vi "Process.vi"(8 "error in (no error)":errorcluster, 11 "qbus in":refnum<class "Qbus.lvclass">) -> (0 "error out":errorcluster)   [LabVIEW 2017, in "TraceLogger.lvlib"]
doc: "This process receives tracepoint instances, writes them to temporary log files on the device disk, and forwards them to the TracePoint Synchronizer process. Separately, the TracePoint Synchronizer process sends tracepoint instances to NI InsightCM Server and informs Tracelogger process when the list of enabled tracepoints changes."
uses:
  <vilib>/addons/TraceLogger/TraceLogger.lvlib
  <vilib>/addons/Qbus/Qbus.lvclass
  <vilib>/addons/TraceLogger/controls/config.ctl
  <vilib>/addons/TraceLogger/controls/LogTracepoint.ctl
  <vilib>/addons/TimerProcess/controls/taskType.ctl
  <vilib>/addons/TimerProcess/TimerProcess.lvlib
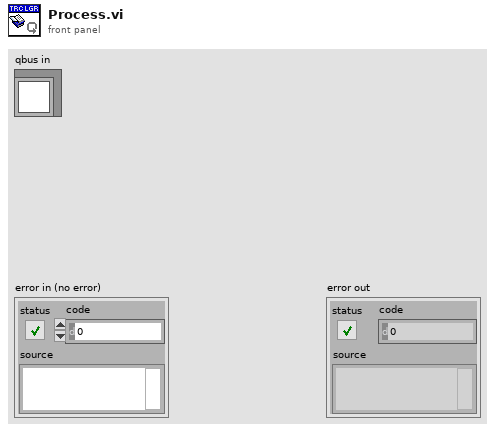
[diagram p1: front panel]
types:
  T1 = typedef "TraceLogger.lvlib/config.ctl" = cluster{"log dir":path, "tracepoints dir":path, "BufferQ":refnum<queue>}
  T2 = typedef "TraceLogger.lvlib/LogTracepoint.ctl" = cluster{"tracepoint":string, "log string":string}
  T3 = typedef "TimerProcess.lvlib/taskType.ctl" = enum16{"single", "repeat"}
  T4 = typedef "TracpointDirectories.ctl" = cluster{"log directory":path, "tracpoint directory":path}
  T5 = typedef "TraceLogger.lvlib/TracepointConfig.ctl" = cluster{"name":string, "enabled":bool}
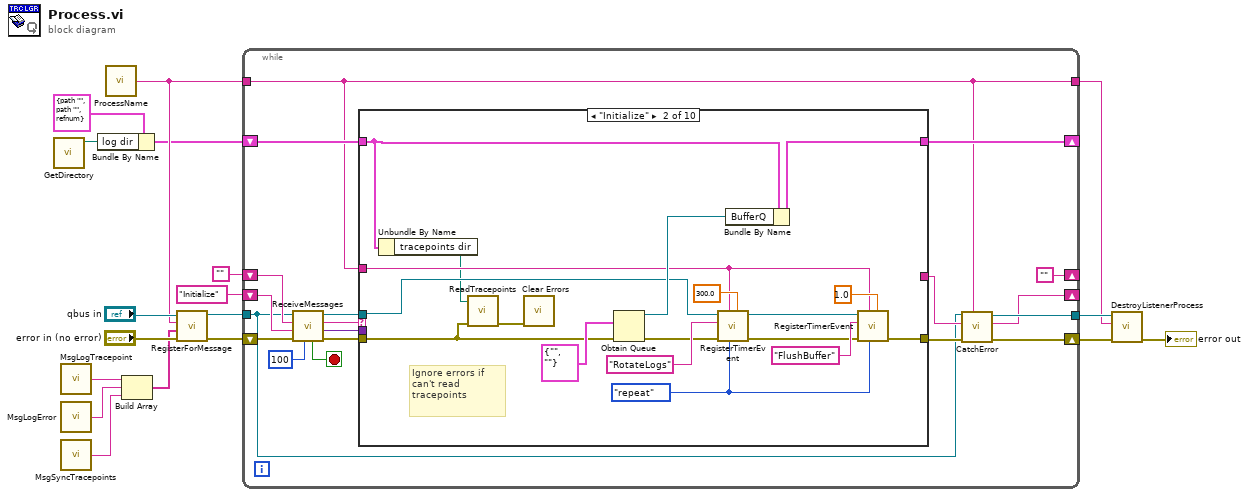
[diagram p0: block diagram]
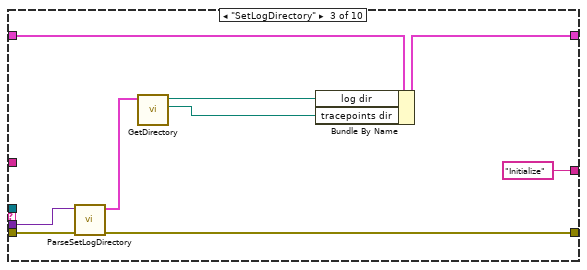
[diagram p3: hidden frame]
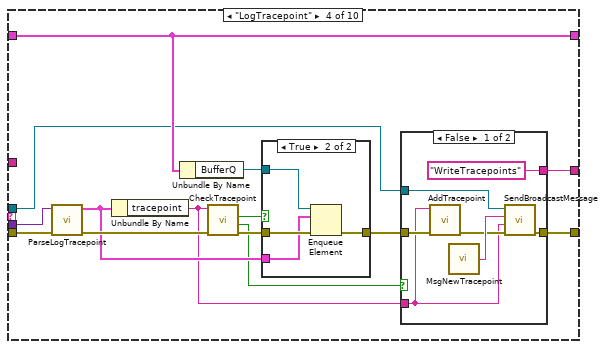
[diagram p4: hidden frame]
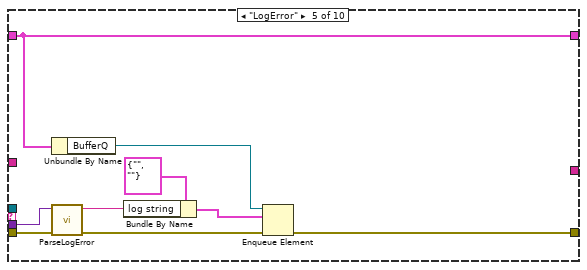
[diagram p7: hidden frame]
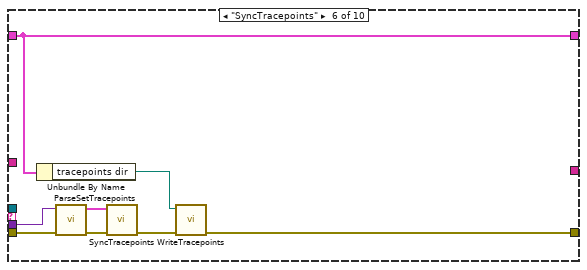
[diagram p8: hidden frame]
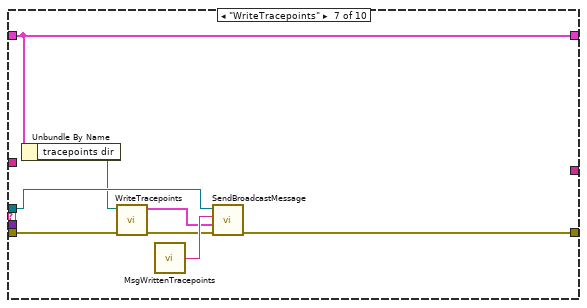
[diagram p9: hidden frame]
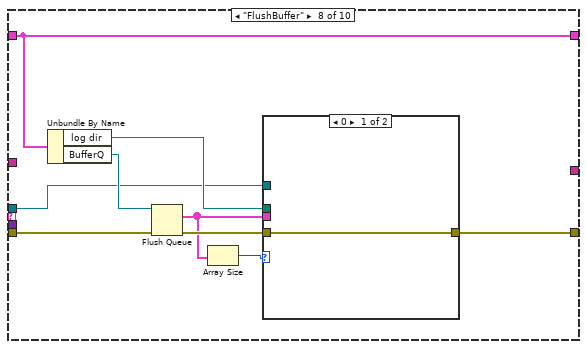
[diagram p10: hidden frame]
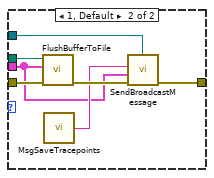
[diagram p11: hidden frame]
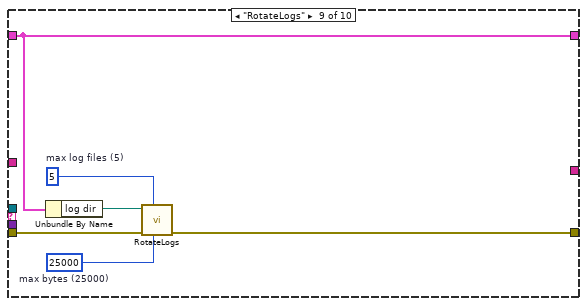
[diagram p12: hidden frame]
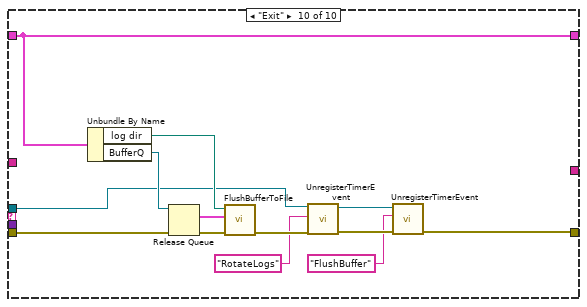
[diagram p13: hidden frame]
diagram:
  n1 = call <vilib>:"GetDirectory.vi"() -> ("log directory"=w4:path)  [unwired: 10 in, 1 out]
  n2 = call <vilib>:"MsgLogTracepoint.vi"() -> ("message name"=w2:string)  [unwired: 5 in]
  n3 = call <vilib>:"MsgLogError.vi"() -> ("message name"=w1:string)  [unwired: 5 in]
  n4 = call <vilib>:"MsgSyncTracepoints.vi"() -> ("message name"=w3:string)  [unwired: 5 in]
  n5 = Bundle By Name(cluster=T1 {"log dir"=path "", "tracepoints dir"=path "", "BufferQ"=refnum} ("config"), "log dir"=w4) -> (w5:T1)
  n6 = call <vilib>:"ProcessName.vi"() -> ("process name"=w8:string)  [unwired: 5 in]
  n7 = Build Array(w2, w1, w3) -> (w7:string[])
  n8 = call <vilib>:"RegisterForMessage.vi"("error in (no error)"="error in (no error)", "message names"=w7, "process name"=w8, "Qbus in"="qbus in") -> ("error in (no error)"=w17:errorcluster, "Qbus out"=w16:refnum<class "Qbus.lvclass">)  [unwired: 6 in]
  n9 = while {
    shift-right: [""] -> _
    shift-left: "" -> [w35]
    tunnel: w16 -> [w21]
    tunnel: w8 -> [w24]
    tunnel: [w26] -> w13
    tunnel: [w24] -> w12
    shift-right: [w25] -> _
    shift-left: "Initialize" -> [w30]
    shift-right: [w28] -> _
    shift-left: w5 -> [w29]
    shift-right: [w27] -> w15
    shift-left: w17 -> [w37]
    stop <- w36 stop-if-true
    n10 = call <vilib>:"ReceiveMessages.vi"("timeout(100)"=100, "error in (no error)"=w37, "priority action"=w30, "default action"=w35, "qbus in"=w21) -> ("error out"=w34:errorcluster, "message value"=w31:variant, "action"=w20:string, "qbus out"=w32:refnum<class "Qbus.lvclass">, "exit"=w36:bool)  [unwired: 2 in]
    n11 = case shown="\"Initialize\"" w20 {
      tunnel: w34 -> [w39 w42 w66 w80 w102 w110 w117 w126 w141 w151]
      tunnel: w32 -> [_ w43 _ w70 _ _ w114 w122 _ w145]
      tunnel: [w39 w45 w65 w69 w98 w103 w115 w121 w140 w146] -> w22
      tunnel: w31 -> [_ _ w64 w79 w101 w109 _ _ _ _]
      tunnel: w29 -> [w38 w41 w63 w77 w100 w106 w118 w127 w139 w150]
      tunnel: [w38 w55 w62 w77 w100 w106 w118 w127 w139 w150] -> w28
      tunnel: w24 -> [_ w44 _ _ _ _ _ _ _ _]
      tunnel: [_ _ "Initialize" w67 _ _ _ _ _ _] -> w23
      frame "", Default {
      }
      frame "Initialize" {
        w51 = taskType."repeat" ("type")
        # "Ignore errors if can't read tracepoints"
        n12 = Unbundle By Name(w41) -> ("tracepoints dir"=w40:path)
        n13 = call <vilib>:"ReadTracepoints.vi"("error in (no error)"=w42, "log dir"=w40) -> ("error out"=w57:errorcluster)  [unwired: 9 in]
        n14 = call <vilib>:"Clear Errors.vi"("error in (no error)"=w57) -> ()  [unwired: 5 in, 2 out]
        n15 = Obtain Queue(element data type=T2 {"tracepoint"="", "log string"=""} ("Buffer"), error in (no error)=w42) -> (queue out=w54:refnum<queue>, error out=w46:errorcluster)  [unwired: 3 in, 1 out]
        n16 = call <vilib>:"RegisterTimerEvent.vi"("interval (sec)"=300.0, "type"=w51, "process name"=w44, "error in (no error)"=w46, "callback action"="RotateLogs" ("CallBackLoop"), "qbus in"=w43) -> ("error out"=w49:errorcluster, "qbus out"=w53:refnum<class "Qbus.lvclass">)  [unwired: 4 in]
        n17 = Bundle By Name(cluster=w41, "BufferQ"=w54) -> (w55:T1)
        n18 = call <vilib>:"RegisterTimerEvent.vi"("interval (sec)"=1.0, "type"=w51, "process name"=w44, "error in (no error)"=w49, "callback action"="FlushBuffer" ("CallBackLoop"), "qbus in"=w53) -> ("error out"=w45:errorcluster)  [unwired: 4 in, 1 out]
      }
      frame "SetLogDirectory" {
        n19 = call <vilib>:"ParseSetLogDirectory.vi"("error in (no error)"=w66, "message body"=w64) -> ("error out"=w65:errorcluster, "tracepoint directories"=w60:T4)  [unwired: 8 in]
        n20 = call <vilib>:"GetDirectory.vi"("tracpoint directories"=w60) -> ("tracepoint directory"=w58:path, "log directory"=w59:path)  [unwired: 9 in]
        n21 = Bundle By Name(cluster=w63, "log dir"=w59, "tracepoints dir"=w58) -> (w62:T1)
      }
      frame "LogTracepoint" {
        n22 = call <vilib>:"ParseLogTracepoint.vi"("error in (no error)"=w80, "message body"=w79) -> ("error out"=w78:errorcluster, "tracelog"=w73:T2)  [unwired: 8 in]
        n23 = Unbundle By Name(w73) -> ("tracepoint"=w68:string)
        n24 = Unbundle By Name(w77) -> ("BufferQ"=w74:refnum<queue>)
        n25 = call <vilib>:"CheckTracepoint.vi"("error in (no error)"=w78, "tracepoint"=w68) -> ("error out"=w75:errorcluster, "found"=w71:bool, "enabled"=w76:bool)  [unwired: 7 in]
        n26 = case shown="True" w76 {
          tunnel: w75 -> [w89 w93]
          tunnel: w74 -> [_ w92]
          tunnel: w73 -> [_ w91]
          tunnel: [w89 w90] -> w72
          frame False {
          }
          frame True {
            n27 = Enqueue Element(queue=w92, element=w91, error in (no error)=w93) -> (error out=w90:errorcluster)  [unwired: 1 in, 2 out]
          }
        }
        n28 = case shown="False" w71 {
          tunnel: w72 -> [w83 w88]
          tunnel: w70 -> [w87 _]
          tunnel: [w85 w88] -> w69
          tunnel: w68 -> [w81 _]
          tunnel: ["WriteTracepoints" _] -> w67
          frame False {
            n29 = call <vilib>:"AddTracepoint.vi"("error in (no error)"=w83, "tracepoint"=w81) -> ("error out"=w82:errorcluster)  [unwired: 9 in]
            n30 = call <vilib>:"MsgNewTracepoint.vi"() -> ("message name"=w86:string)  [unwired: 5 in]
            n31 = call <vilib>:"SendBroadcastMessage.vi"("error in (no error)"=w82, "message value"=w81, "message name"=w86, "Qbus in"=w87) -> ("error in (no error)"=w85:errorcluster)  [unwired: 6 in, 1 out]
          }
          frame True {
          }
        }
      }
      frame "LogError" {
        n32 = Unbundle By Name(w100) -> ("BufferQ"=w99:refnum<queue>)
        n33 = call <vilib>:"ParseLogError.vi"("error in (no error)"=w102, "message body"=w101) -> ("error out"=w97:errorcluster, "error string"=w95:string)  [unwired: 8 in]
        n34 = Bundle By Name(cluster=T2 {"tracepoint"="", "log string"=""} ("element"), "log string"=w95) -> (w94:T2)
        n35 = Enqueue Element(queue=w99, element=w94, error in (no error)=w97) -> (error out=w98:errorcluster)  [unwired: 1 in, 2 out]
      }
      frame "SyncTracepoints" {
        n36 = Unbundle By Name(w106) -> ("tracepoints dir"=w105:path)
        n37 = call <vilib>:"ParseSetTracepoints.vi"("error in (no error)"=w110, "message body"=w109) -> ("error out"=w108:errorcluster, "tracepoints"=w107:T5[])  [unwired: 8 in]
        n38 = call <vilib>:"SyncTracepoints.vi"("error in (no error)"=w108, "new tracepoints"=w107) -> ("error out"=w104:errorcluster)  [unwired: 9 in]
        n39 = call <vilib>:"WriteTracepoints.vi"("error in (no error)"=w104, "log dir"=w105) -> ("error out"=w103:errorcluster)  [unwired: 8 in, 1 out]
      }
      frame "WriteTracepoints" {
        n40 = Unbundle By Name(w118) -> ("tracepoints dir"=w113:path)
        n41 = call <vilib>:"WriteTracepoints.vi"("error in (no error)"=w117, "log dir"=w113) -> ("error out"=w111:errorcluster, "tracepoints"=w112:T5[])  [unwired: 8 in]
        n42 = call <vilib>:"MsgWrittenTracepoints.vi"() -> ("message name"=w116:string)  [unwired: 5 in]
        n43 = call <vilib>:"SendBroadcastMessage.vi"("error in (no error)"=w111, "message value"=w112, "message name"=w116, "Qbus in"=w114) -> ("error in (no error)"=w115:errorcluster)  [unwired: 6 in, 1 out]
      }
      frame "FlushBuffer" {
        n44 = Unbundle By Name(w127) -> ("log dir"=w123:path, "BufferQ"=w125:refnum<queue>)
        n45 = Flush Queue(queue=w125, error in (no error)=w126) -> (remaining elements=w120:T2[], error out=w124:errorcluster)  [unwired: 1 out]
        n46 = Array Size(array=w120) -> (size(s)=w119:i32)
        n47 = case shown="0" w119 {
          tunnel: w124 -> [w128 w135]
          tunnel: w123 -> [_ w134]
          tunnel: w122 -> [_ w132]
          tunnel: [w128 w130] -> w121
          tunnel: w120 -> [_ w129]
          frame 0 {
          }
          frame 1, Default {
            n48 = call <vilib>:"FlushBufferToFile.vi"("error in (no error)"=w135, "tracepoints"=w129, "log dir"=w134) -> ("error out"=w133:errorcluster)  [unwired: 8 in]
            n49 = call <vilib>:"MsgSaveTracepoints.vi"() -> ("message name"=w131:string)  [unwired: 5 in]
            n50 = call <vilib>:"SendBroadcastMessage.vi"("error in (no error)"=w133, "message value"=w129, "message name"=w131, "Qbus in"=w132) -> ("error in (no error)"=w130:errorcluster)  [unwired: 6 in, 1 out]
          }
        }
      }
      frame "RotateLogs" {
        w136 = 25000  # max bytes (25000)
        w137 = 5  # max log files (5)
        n51 = Unbundle By Name(w139) -> ("log dir"=w138:path)
        n52 = call <vilib>:"RotateLogs.vi"("max bytes (25000)"=w136, "max log files (5)"=w137, "error in (no error)"=w141, "log dir"=w138) -> ("error out"=w140:errorcluster)  [unwired: 7 in]
      }
      frame "Exit" {
        n53 = Unbundle By Name(w150) -> ("log dir"=w154:path, "BufferQ"=w153:refnum<queue>)
        n54 = Release Queue(queue=w153, error in (no error)=w151) -> (remaining elements=w152:T2[], error out=w149:errorcluster)  [unwired: 1 in, 1 out]
        n55 = call <vilib>:"FlushBufferToFile.vi"("error in (no error)"=w149, "tracepoints"=w152, "log dir"=w154) -> ("error out"=w148:errorcluster)  [unwired: 8 in]
        n56 = call <vilib>:"UnregisterTimerEvent.vi"("error in (no error)"=w148, "timer task name"="RotateLogs" ("CallBackLoop"), "qbus in"=w145) -> ("error out"=w147:errorcluster, "qbus out"=w144:refnum<class "Qbus.lvclass">)  [unwired: 7 in]
        n57 = call <vilib>:"UnregisterTimerEvent.vi"("error in (no error)"=w147, "timer task name"="FlushBuffer" ("CallBackLoop"), "qbus in"=w144) -> ("error out"=w146:errorcluster)  [unwired: 7 in, 1 out]
      }
    }
    n58 = call <vilib>:"CatchError.vi"("source"=w24, "error in (no error)"=w22, "next action in"=w23, "Qbus in"=w21) -> ("error out"=w27:errorcluster, "next action out"=w25:string, "Qbus out"=w26:refnum<class "Qbus.lvclass">)  [unwired: 5 in]
  }
  n59 = call <vilib>:"DestroyListenerProcess.vi"("error in (no error)"=w15, "process name"=w12, "Qbus in"=w13) -> ("error in (no error)"=→"error out":errorcluster)  [unwired: 7 in, 1 out]
